vi "read PCROS.vi"(8 "error in (no error)":errorcluster, 11 "ASI stage":T1) -> (0 "error out":errorcluster, 3 "ASI stage out":T1)   [LabVIEW 2010]
uses:
  stage properties.ctl
panel:
  out "Raw receive buffer":string
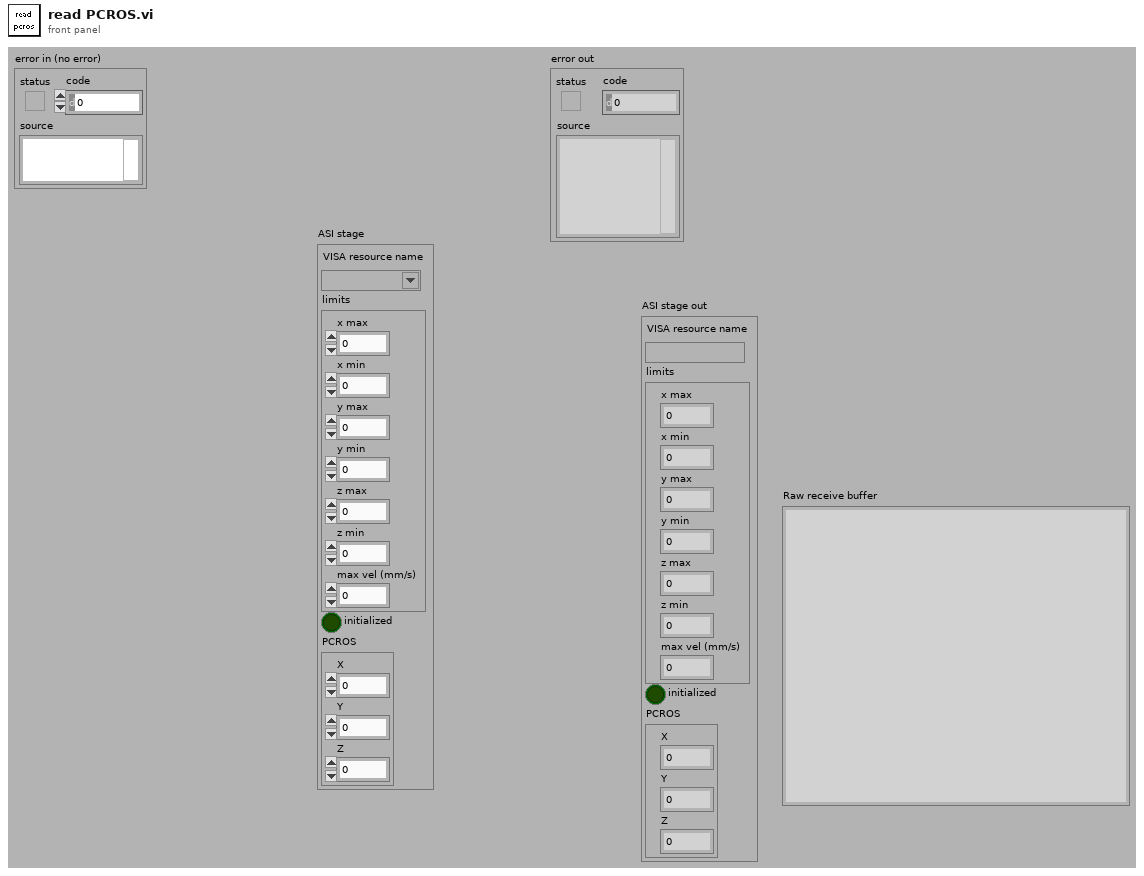
[diagram p1: front panel]
types:
  T1 = typedef "stage properties.ctl" = cluster{"VISA resource name":refnum<visa-resource-name>, "limits":cluster{"x max":dbl, "x min":dbl, "y max":dbl, "y min":dbl, "z max":dbl, "z min":dbl, "max vel (mm/s)":dbl}, "initialized":bool, "PCROS":cluster{"X":dbl, "Y":dbl, "Z":dbl}}
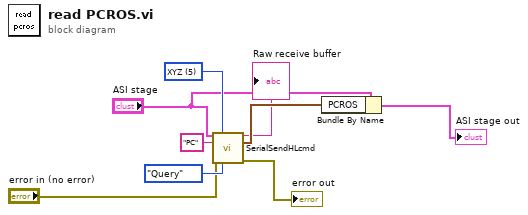
[diagram p0: block diagram]
diagram:
  w8 = u16 5 items=["No axis", "X", "Y", "Z", "XY", "XYZ"] ("Axis configuration")
  n1 = call "SerialSendHLcmd.vi"("ASI stage"="ASI stage", "Axis configuration"=w8, "Command"="PC", "error in (no error)"="error in (no error)", "Command type"=enum16{"Query", "Where", "Imperative", "DU Y"}."Query") -> ("Raw receive buffer"=→"Raw receive buffer":string, "data out"=w5:cluster{"X out":dbl, "Y out":dbl, "Z out":dbl}, "error out"=→"error out":errorcluster)  [unwired: 8 in]
  n2 = Bundle By Name(cluster="ASI stage", "PCROS"=w5) -> (→"ASI stage out":T1)
